vi "SetCellStyles.vi"(4 "Column":i32, 6 "Row":i32, 8 "error in (no error)":errorcluster, 10 "CellStyle.lvclass":refnum<class "CellStyle.lvclass">, 11 "DataGridView in":refnum<class "DataGridView.lvclass">) -> (0 "error out":errorcluster, 3 "DataGridView out":refnum<class "DataGridView.lvclass">)   [LabVIEW 2020, in "DataGrid.lvlib" / "DataGridView.lvclass"]
doc: "Applies a cell style to any cell, by row and column. If the row is set to -1, it will apply to the column headers.\n\nUse this sparingly, as it can have a very negative effect on performance. Instead, use the DefaultCellStyle and AlternatingRowsDefaultCellStyle"
uses:
  DataGridView.lvclass
  CellStyle/CellStyle.lvclass
  CellStyle/CellStyle.lvclass/CellStyle.ctl
  DataGridView.lvclass/DataGridView.ctl
  System.Windows.Forms
  CellStyle/Properties/Read cellStyle.vi
  Properties/Read DataGridView.vi
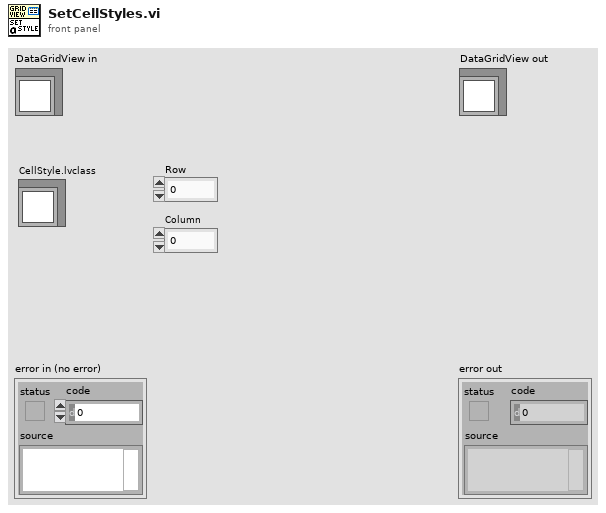
[diagram p1: front panel]
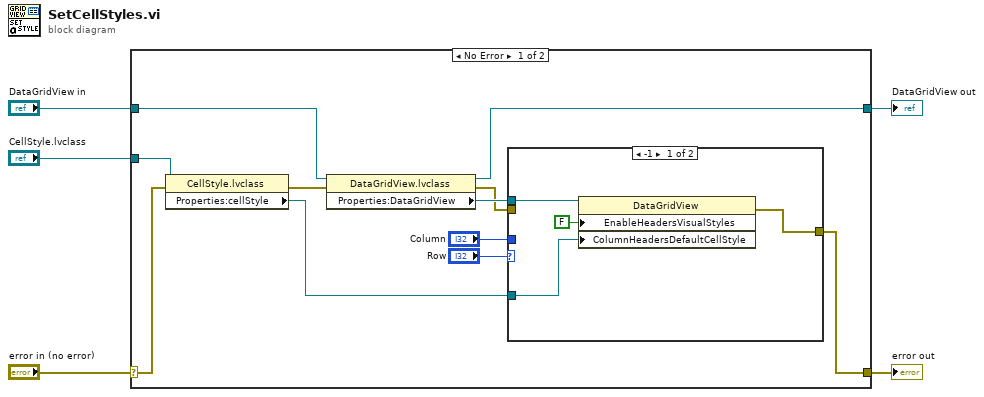
[diagram p0: block diagram]
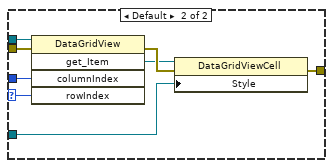
[diagram p2: hidden frame]
diagram:
  n1 = case shown="No Error" "error in (no error)" {
    selector: "error in (no error)" -> [w15 w30]
    tunnel: [w13 w30] -> w4
    tunnel: [w6 w29] -> w2
    tunnel: "DataGridView in" -> [w7 w29]
    tunnel: "CellStyle.lvclass" -> [w16 _]
    frame No Error {
      n2 = property class="CellStyle.lvclass"(reference=w16, error in=w15) -> (error out=w14:errorcluster, "Properties:cellStyle"=w9:refnum<k24>)  [unwired: 1 out]
      n3 = property class="DataGridView.lvclass"(reference=w7, error in=w14) -> (reference out=w6:refnum<class "DataGridView.lvclass">, error out=w10:errorcluster, "Properties:DataGridView"=w12:refnum<k24>)
      n4 = case shown="-1" "Row" {
        selector: "Row" -> [_ w21]
        tunnel: [w19 w28] -> w13
        tunnel: w12 -> [w20 w27]
        tunnel: "Column" -> [_ w26]
        tunnel: w10 -> [_ w25]
        tunnel: w9 -> [w18 w22]
        frame -1 {
          n5 = property class="DataGridView"(reference=w20, "EnableHeadersVisualStyles"=FALSE, "ColumnHeadersDefaultCellStyle"=w18) -> (error out=w19:errorcluster)  [unwired: 1 in, 1 out]
        }
        frame Default {
          n6 = invoke class="DataGridView" method="get_Item"(reference=w27, error in=w25, "columnIndex"=w26, "rowIndex"=w21) -> (error out=w24:errorcluster, "get_Item"=w23:refnum<k24>)  [unwired: 1 in, 3 out]
          n7 = property class="DataGridViewCell"(reference=w23, error in=w24, "Style"=w22) -> (error out=w28:errorcluster)  [unwired: 1 out]
        }
      }
    }
    frame Error {
    }
  }
  "error out" <- w4
  "DataGridView out" <- w2
